vi "Image Threshold.vi"() -> ()   [LabVIEW 2014]
doc: "This example illustrates different thresholding algorithms. Local thresholding calculates local statistics for each pixel in an image. Based on the calculation result, the algorithm categorizes the pixel as part of a particle or the background. Automatic thresholding uses the histogram of an image to compute a single threshold value for the entire image. Manual thresholding uses a specified range of values to compute a threshold value for the image. Refer to the NI Vision Concepts Manual for more information about thresholding algorithms."
uses:
  <vilib>/vision/NI_Vision_Development_Module.lvlib
panel:
  in  "Type":T1(tab)
  in  "Local":T2={"Object Type"=1, "Method"=1, "Niblack Deviation Factor"=1.0, "Window"={"Width"=160, "Height"=160}} {"Niblack Deviation Factor" min=0.0 max=1.0 step=0.1 format="%.2f"; "Method" items=["Niblack", "Background Correction"]; "Object Type" items=["Bright Objects", "Dark Objects"]}
  in  "Automatic":cluster{"Object Type":u32, "Method":i32}={"Object Type"=1, "Method"=0} {"Method" items=["clustering", "entropy", "metric", "moments", "inter-class variance"]; "Object Type" items=["Bright Objects", "Dark Objects"]}
  in  "Manual":cluster{sgl, sgl}(slide)={0.0, 150.0} caption="Threshold Range" scale=0.0..255.0
  in  "Number of Classes":i32=2 min=2 step=1
  out "Original":T3(plugin-control)
  in  "Stop":bool
  out "Dst":T3(plugin-control)
  # "Overview: Demonstrates how to use different Threshold functions with an unevenly lit LCD display.\nRequirements: Vision Development Software.\nInstructions:\n1. Run the VI.\n2. Click on the different Threshold algorithm tabs to see how each algorithm works. The local threshold is the most robust algorithm when there are lighting variations in the image."
  # "Minimum"
  # "Maximum"
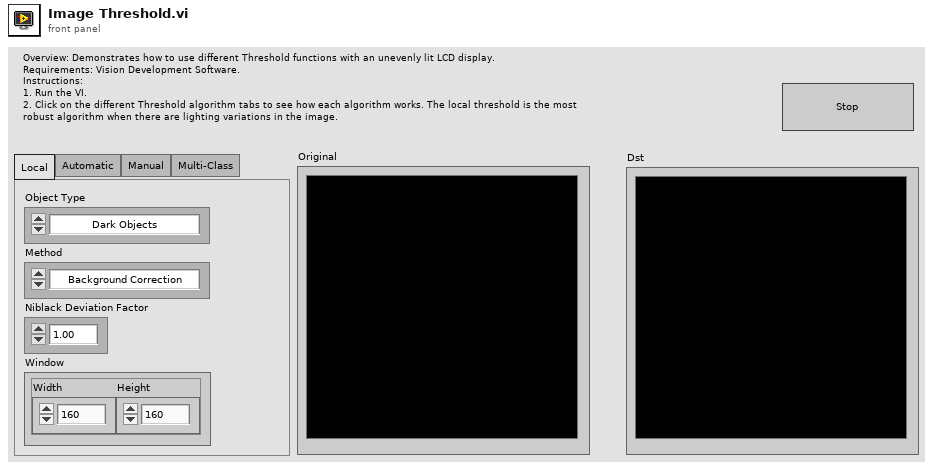
[diagram p1: front panel]
types:
  T1 = enum32{"Local", "Automatic", "Manual", "Multi-Class"}
  T2 = cluster{"Object Type":u32, "Method":u32, "Niblack Deviation Factor":dbl, "Window":cluster{"Width":i32, "Height":i32}}
  T3 = typedef "IMAQ Image.ctl" = refnum<image>
  T4 = cluster{"Lower value":i32, "Upper value":i32, "Replace Value":i32, "Keep/Replace Value (Replace)":bool}[]
  T5 = cluster{"Type":enum32{"Local", "Automatic", "Manual", "Multi-Class"}, "Local":cluster{"Object Type":u32, "Method":u32, "Niblack Deviation Factor":dbl, "Window":cluster{"Width":i32, "Height":i32}}, "Automatic":cluster{"Object Type":u32, "Method":i32}, "Manual":cluster{sgl, sgl}, "Number of Classes":i32}
  T6 = cluster{"Lower value":sgl, "Upper value":sgl, "Replace Value":sgl, "Keep/Replace Value (Replace)":bool}[]
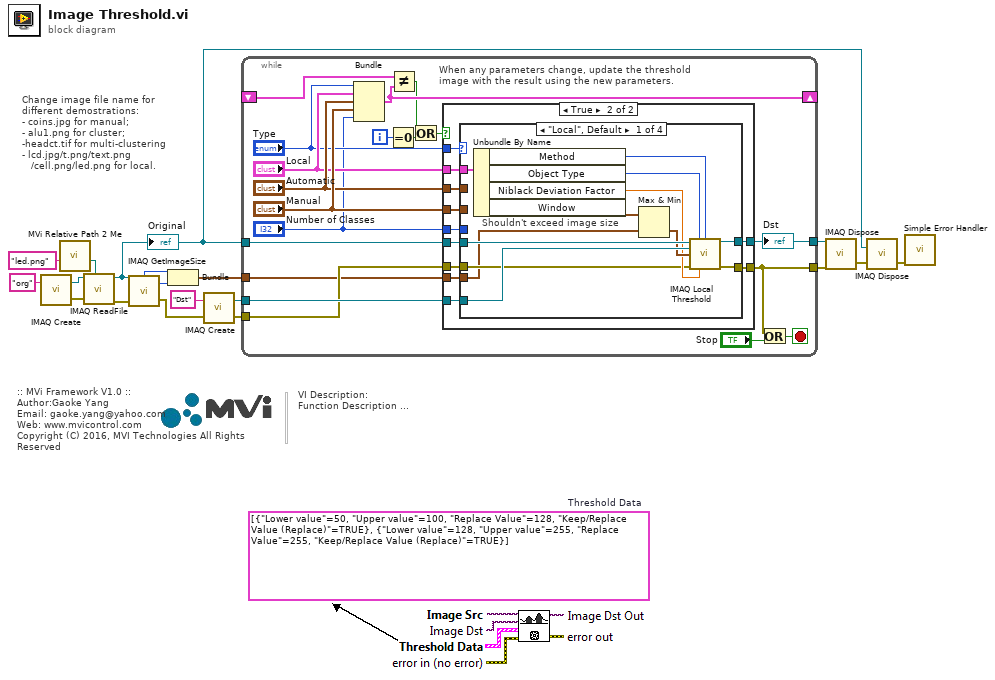
[diagram p0: block diagram]
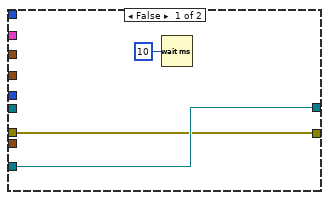
[diagram p2: hidden frame]
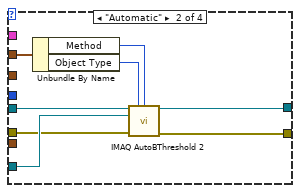
[diagram p3: hidden frame]
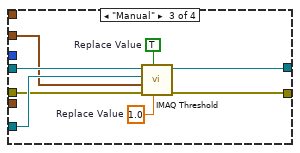
[diagram p4: hidden frame]
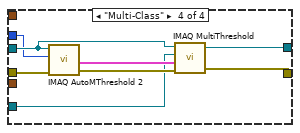
[diagram p5: hidden frame]
diagram:
  (unwired) T4 [{"Lower value"=50, "Upper value"=100, "Replace Value"=128, "Keep/Replace Value (Replace)"=TRUE}, {"Lower value"=128, "Upper value"=255, "Replace Value"=255, "Keep/Replace Value (Replace)"=TRUE}]  # Threshold Data
  # "VI Description:\nFunction Description ..."
  # ":: MVi Framework V1.0 ::\nAuthor:Gaoke Yang\nEmail: gaoke.yang@yahoo.com\nWeb: www.mvicontrol.com\nCopyright (C) 2016, MVI Technologies All Rights Reserved"
  # "Change image file name for \ndifferent demostrations:\n- coins.jpg for manual;\n- alu1.png for cluster;\n-headct.tif for multi-clustering\n- lcd.jpg/t.png/text.png\n   /cell.png/led.png for local."
  n1 = call "IMAQ Create"("Image Name"="org") -> ("New Image"=w14:T3, "error out"=w13:errorcluster)  [unwired: 4 in]
  n2 = call "MVi Relative Path 2 Me.vi"("Relative Path"="led.png" ("name or relative path")) -> ("Appended Dir"=w1:path)  [unwired: 5 in, 1 out]
  n3 = call "IMAQ ReadFile"("File Path"=w1, "error in (no error)"=w13, "Image"=w14) -> ("error out"=w15:errorcluster, "Image Out"=w5:T3)  [unwired: 4 in, 3 out]
  "Original" <- w5
  n4 = call "IMAQ GetImageSize"("Image"=w5, "error in (no error)"=w15) -> ("Y Resolution"=w10:i32, "X Resolution"=w11:i32, "error out"=w12:errorcluster)  [unwired: 2 in]
  n5 = Bundle("X Resolution"=w11, "Y Resolution"=w10) -> (w3:cluster{"X Resolution":i32, "Y Resolution":i32})  [unwired: 1 in]
  n6 = call "IMAQ Create"("Image Name"="Dst", "error in (no error)"=w12) -> ("New Image"=w18:T3, "error out"=w9:errorcluster)  [unwired: 3 in]
  n7 = while {
    tunnel: w5 -> [w37]
    tunnel: w18 -> [w36]
    tunnel: w9 -> [w27]
    shift-right: [w31] -> _
    shift-left: _ -> [w30]
    tunnel: [w21] -> w7
    tunnel: [w28] -> w8
    tunnel: w3 -> [w26]
    i -> [w25]
    stop <- w29 stop-if-true
    # "When any parameters change, update the threshold image with the result using the new parameters."
    n8 = Bundle("Type"="Type", "Local"="Local", "Automatic"="Automatic", "Manual"="Manual", "Number of Classes"="Number of Classes") -> (w31:T5)  [unwired: 1 in]
    n9 = Equal To 0?(x=w25) -> (x = 0?=w24:bool)
    n10 = Not Equal?(x=w30, y=w31) -> (x != y?=w22:bool)
    n11 = Or(x=w22, y=w24) -> (x .or. y?=w23:bool)
    n12 = case shown="True" w23 {
      tunnel: w37 -> [_ w51]
      tunnel: w36 -> [w40 w50]
      tunnel: [w40 w49] -> w28
      tunnel: "Manual" -> [_ w48]
      tunnel: "Automatic" -> [_ w47]
      tunnel: "Local" -> [_ w46]
      tunnel: "Type" -> [_ w45]
      tunnel: [w38 w44] -> w21
      tunnel: w27 -> [w38 w43]
      tunnel: w26 -> [_ w42]
      tunnel: "Number of Classes" -> [_ w41]
      frame False {
        n13 = Wait (ms)(milliseconds to wait=u32 10) -> ()  [unwired: 1 out]
      }
      frame True {
        n14 = case shown="\"Local\", Default" w45 {
          tunnel: w51 -> [w63 w71 w79 w82]
          tunnel: w50 -> [w62 w70 w78 w83]
          tunnel: [w61 w69 w77 w81] -> w49
          tunnel: w46 -> [w60 _ _ _]
          tunnel: w47 -> [_ w68 _ _]
          tunnel: [w54 w67 w75 w85] -> w44
          tunnel: w48 -> [_ _ w76 _]
          tunnel: w43 -> [w53 w64 w74 w87]
          tunnel: w42 -> [w52 _ _ _]
          tunnel: w41 -> [_ _ _ w80]
          frame "Local", Default {
            # "Shouldn't exceed image size"
            n15 = Unbundle By Name(w60) -> ("Method"=w58:u32, "Object Type"=w57:u32, "Niblack Deviation Factor"=w56:dbl, "Window"=w55:cluster{"Width":i32, "Height":i32})
            n16 = Max & Min(x=w55, y=w52) -> (min(x,y)=w59:cluster{i32, i32})  [unwired: 1 out]
            n17 = call "IMAQ Local Threshold"("Image Src"=w63, "Look For (Bright Objects)"=w57, "Method (Niblack)"=w58, "Image Dst"=w62, "Window Size (32x32)"=w59, "error in (no error)"=w53, "Niblack Deviation Factor (0.2)"=w56) -> ("Image Dst Out"=w61:T3, "error out"=w54:errorcluster)  [unwired: 7 in]
          }
          frame "Automatic" {
            n18 = Unbundle By Name(w68) -> ("Method"=w66:i32, "Object Type"=w65:u32)
            n19 = call "IMAQ AutoBThreshold 2"("Image Src"=w71, "Look For (Bright Objects)"=w65, "Method (clustering)"=w66, "Image Dst"=w70, "error in (no error)"=w64) -> ("Image Dst Out"=w69:T3, "error out"=w67:errorcluster)  [unwired: 8 in, 1 out]
          }
          frame "Manual" {
            w73 = sgl 1.0  # Replace Value
            w72 = TRUE  # Replace Value
            n20 = call "IMAQ Threshold"("Replace Value"=w73, "Keep/Replace Value (Replace)"=w72, "error in (no error)"=w74, "Range"=w76, "Image Dst"=w78, "Image Src"=w79) -> ("error out"=w75:errorcluster, "Image Dst Out"=w77:T3)  [unwired: 4 in]
          }
          frame "Multi-Class" {
            n21 = call "IMAQ AutoMThreshold 2"("error in (no error)"=w87, "Number of Classes"=w80, "Image"=w82) -> ("error out"=w86:errorcluster, "Threshold Data out"=w84:T6)  [unwired: 1 in, 1 out]
            n22 = call "IMAQ MultiThreshold"("error in (no error)"=w86, "Threshold Data"=w84, "Image Dst"=w83, "Image Src"=w82) -> ("error out"=w85:errorcluster, "Image Dst Out"=w81:T3)  [unwired: 1 in]
          }
        }
      }
    }
    "Dst" <- w28
    n23 = Or(x=w21, y="Stop") -> (x .or. y?=w29:bool)
  }
  n24 = call "IMAQ Dispose"("Image"=w8, "error in (no error)"=w7) -> ("error out"=w6:errorcluster)  [unwired: 4 in]
  n25 = call "IMAQ Dispose"("Image"=w5, "error in (no error)"=w6) -> ("error out"=w4:errorcluster)  [unwired: 4 in]
  n26 = call <vilib>:"Simple Error Handler.vi"("error in (no error)"=w4) -> ()  [unwired: 4 in, 5 out]
